vi "Get Wfm Refs.vi"(8 "Error in":errorcluster, 11 "Device Ref in":T2 format="%.0x") -> (0 "Error out":errorcluster, 1 "Results Wfm Data Refs":T1[](array[typedef]), 2 "Source Wfm Data Refs":T1[](array[typedef]), 3 "Device Ref out":T2=18446744073709551615 format="%.0x")   [LabVIEW 2020, in "Waveform-Processing-Custom-Device System Explorer.lvlib"]
uses:
  Waveform-Processing-Custom-Device System Explorer.lvlib
  <vilib>/NI VeriStand/Custom Device API/Custom Device Item Ref.ctl
  <vilib>/NI VeriStand/Custom Device API/Waveform Data Reference.ctl
  Shared/Constants.vi
  <vilib>/NI VeriStand/Custom Device API/Get Item Property (Dependent Node Pointer).vi
  <vilib>/NI VeriStand/Custom Device API/Custom Device API.lvlib
  Shared/Waveform-Processing-Custom-Device Shared.lvlib
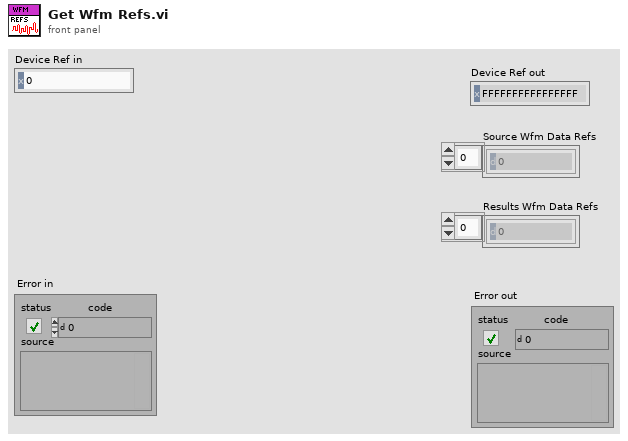
[diagram p1: front panel]
types:
  T1 = typedef "Custom Device API.lvlib/Waveform Data Reference.ctl" = i32
  T2 = typedef "Custom Device API.lvlib/Custom Device Item Ref.ctl" = u64
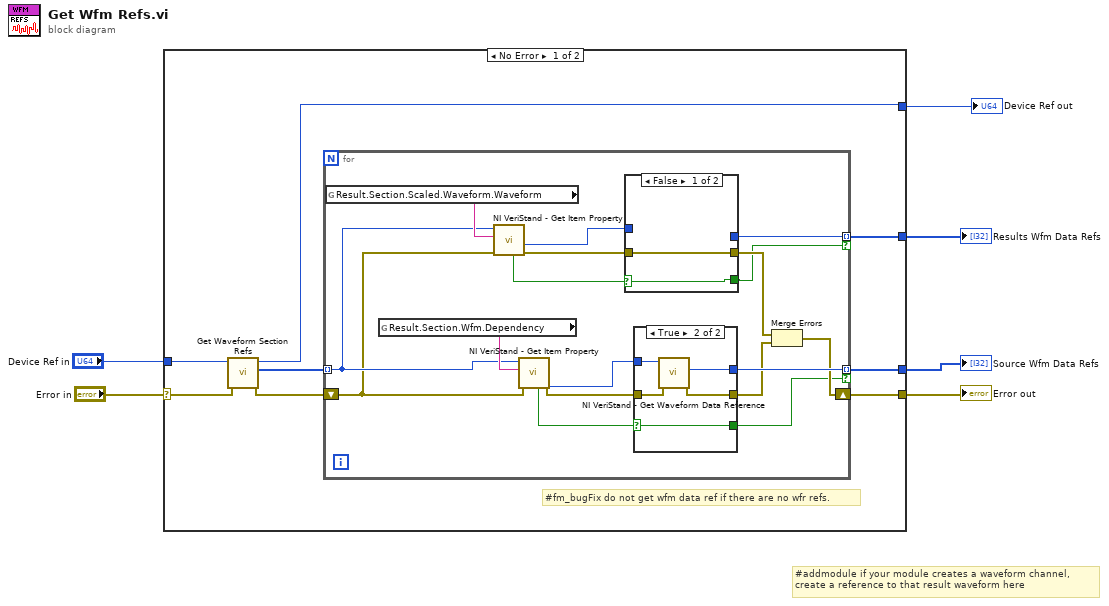
[diagram p0: block diagram]
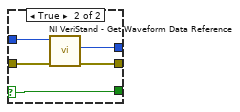
[diagram p3: hidden frame]
diagram:
  # "#addmodule if your module creates a waveform channel,\ncreate a reference to that result waveform here"
  n1 = case shown="No Error" "Error in" {
    selector: "Error in" -> [w14 w47]
    tunnel: [w7 w47] -> w5
    tunnel: "Device Ref in" -> [w13 w46]
    tunnel: [w10 w46] -> w3
    tunnel: [w9 _] -> w2
    tunnel: [w8 _] -> w1
    frame No Error {
      # "#fm_bugFix do not get wfm data ref if there are no wfr refs."
      n2 = call "Get Waveform Section Refs.vi"("Error in"=w14, "Device Ref in"=w13) -> ("Error out"=w12:errorcluster, "Result Section Refs"=w11:T2[], "Device Ref out"=w10:T2)  [unwired: 7 in]
      n3 = for {
        tunnel: w11 -> [w22] mode=indexing
        tunnel: [w28] -> w9 mode=indexing if=w16
        shift-right: [w27] -> w7
        shift-left: w12 -> [w21]
        tunnel: [w19] -> w8 mode=indexing if=w15
        n4 = global read "Constants.vi" "Result.Section.Scaled.Waveform.Waveform"() -> (w23:string)
        n5 = global read "Constants.vi" "Result.Section.Wfm.Dependency"() -> (w31:string)
        n6 = call-poly <vilib>:"NI VeriStand - Get Item Property.vi"("error in (no error)"=w21, "Property Name"=w23, "Item Ref in"=w22) -> ("error out"=w24:errorcluster, "Dependent Node Ref"=w25:T2, "Found"=w18:bool)  [unwired: 5 in, 1 out]
        n7 = call-poly <vilib>:"NI VeriStand - Get Item Property.vi"("error in (no error)"=w21, "Property Name"=w31, "Item Ref in"=w22) -> ("error out"=w30:errorcluster, "Dependent Node Ref"=w29:T2, "Found"=w17:bool)  [unwired: 5 in, 1 out]
        n8 = case shown="False" w18 {
          selector: w18 -> [w40 w41]
          tunnel: w25 -> [_ w45]
          tunnel: w24 -> [w39 w44]
          tunnel: [w39 w43] -> w20
          tunnel: [_ w42] -> w19
          tunnel: [w40 w41] -> w15
          frame False {
          }
          frame True {
            n9 = call <vilib>:"NI VeriStand - Get Waveform Data Reference.vi"("error in (no error)"=w44, "Waveform Ref in"=w45) -> ("error out"=w43:errorcluster, "Waveform Data Reference"=w42:T1)  [unwired: 7 in, 1 out]
          }
        }
        n10 = case shown="True" w17 {
          selector: w17 -> [w32 w34]
          tunnel: w30 -> [w33 w38]
          tunnel: w29 -> [_ w37]
          tunnel: [_ w36] -> w28
          tunnel: [w33 w35] -> w26
          tunnel: [w32 w34] -> w16
          frame False {
          }
          frame True {
            n11 = call <vilib>:"NI VeriStand - Get Waveform Data Reference.vi"("error in (no error)"=w38, "Waveform Ref in"=w37) -> ("error out"=w35:errorcluster, "Waveform Data Reference"=w36:T1)  [unwired: 7 in, 1 out]
          }
        }
        n12 = Merge Errors(w20, w26) -> (w27:errorcluster)
      }
    }
    frame Error {
    }
  }
  "Error out" <- w5
  "Device Ref out" <- w3
  "Source Wfm Data Refs" <- w2
  "Results Wfm Data Refs" <- w1
